vi "VLC exec.vi"(11 "T160 cam url":string=" rtsp://200.131.64.229:554/live2.sdp") -> (2 "tasklist":string, 3 "Opensvlc":bool)   [LabVIEW 2018]
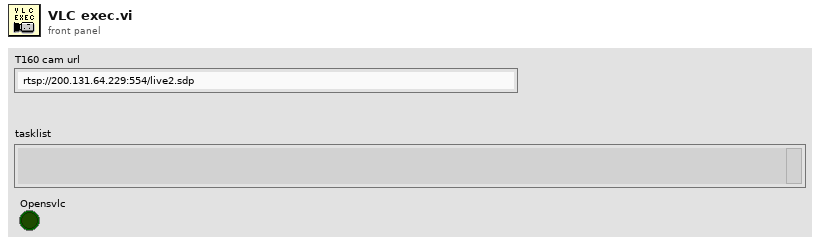
[diagram p1: front panel]
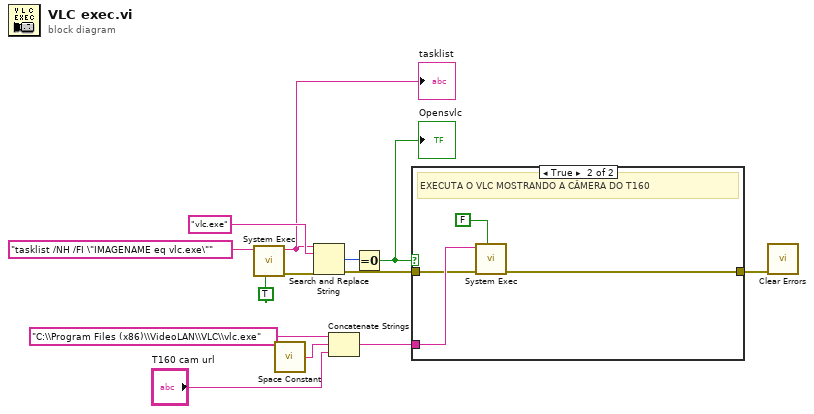
[diagram p0: block diagram]
diagram:
  n1 = call <vilib>:"System Exec.vi"("run minimized? (F)"=TRUE, "command line"="tasklist /NH /FI \"IMAGENAME eq vlc.exe\"") -> ("error out"=w11:errorcluster, "standard output"=w3:string)  [unwired: 6 in, 2 out]
  "tasklist" <- w3
  n2 = call <vilib>:"Space Constant.vi"() -> ("String"=w1:string)
  n3 = Search and Replace String(input string=w3, search string="vlc.exe", error in=w11) -> (number of replacements=w9:i32, error out=w6:errorcluster)  [unwired: 5 in, 2 out]
  n4 = Concatenate Strings("C:\\Program Files (x86)\\VideoLAN\\VLC\\vlc.exe", w1, "T160 cam url") -> (w7:string)
  n5 = Equal To 0?(x=w9) -> (x = 0?=w8:bool)
  "Opensvlc" <- w8
  n6 = case shown="True" w8 {
    tunnel: w7 -> [_ w17]
    tunnel: w6 -> [w14 w16]
    tunnel: [w14 w15] -> w5
    frame False {
    }
    frame True {
      # "EXECUTA O VLC MOSTRANDO A CÂMERA DO T160"
      n7 = call <vilib>:"System Exec.vi"("wait until completion? (T)"=FALSE, "error in (no error)"=w16, "command line"=w17) -> ("error out"=w15:errorcluster)  [unwired: 5 in, 3 out]
    }
  }
  n8 = call <vilib>:"Clear Errors.vi"("error in (no error)"=w5) -> ()  [unwired: 5 in, 2 out]
